vi "Point in Polygon_Classify Quadrant.vi"(6 "tolerance":dbl=1e-09, 8 "Polygon Y":dbl[](array[numeric]), 9 "Polygon X":dbl[](array[numeric]), 10 "y":dbl, 11 "x":dbl) -> (0 "vertex?":bool, 1 "Edge Angle":dbl[](array[numeric]), 2 "Edge Direct":dbl[](array[numeric]), 3 "Edge Quad":i16[](array[numeric]))   [LabVIEW 2020, in "NI_AAL_Geometry.lvlib"]
uses:
  <vilib>/Analysis/NI_AAL_Geometry.lvlib
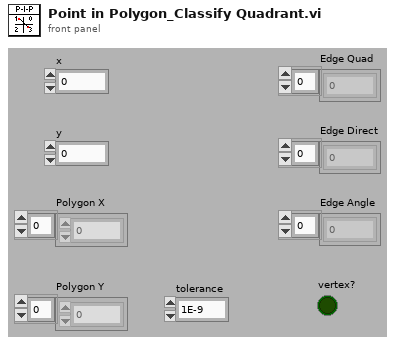
[diagram p1: front panel]
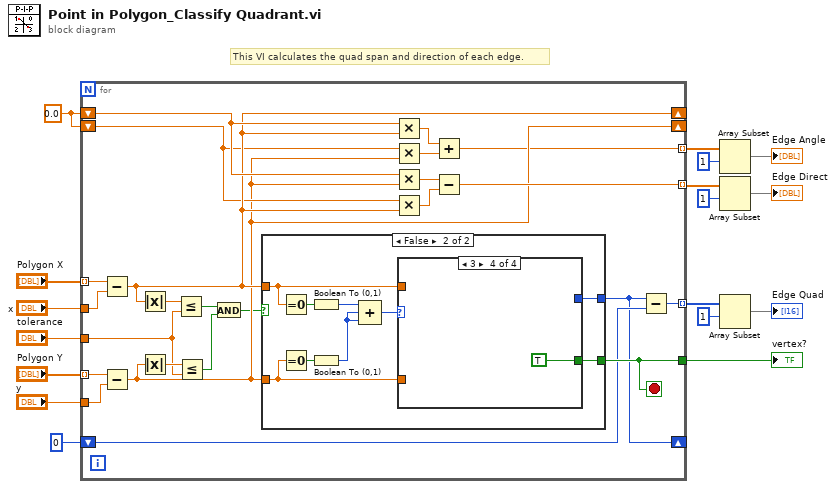
[diagram p0: block diagram]
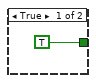
[diagram p2: hidden frame]
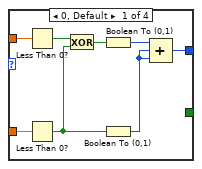
[diagram p3: hidden frame]
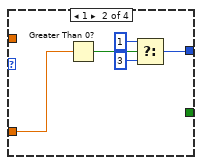
[diagram p4: hidden frame]
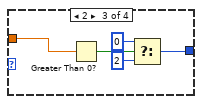
[diagram p5: hidden frame]
diagram:
  w5 = 0.0
  # "This VI calculates the quad span and direction of each edge."
  n1 = for {
    tunnel: "Polygon X" -> [w35] mode=indexing
    tunnel: "Polygon Y" -> [w40] mode=indexing
    tunnel: "x" -> [w41]
    tunnel: "y" -> [w39]
    tunnel: [w38] -> w13
    shift-right: [w18] -> _
    shift-left: i16 0 ("x") -> [w37]
    tunnel: [w36] -> w11 mode=indexing
    shift-right: [w27] -> _
    shift-left: w5 -> [w28]
    shift-right: [w25] -> _
    shift-left: w5 -> [w26]
    tunnel: [w33] -> w8 mode=indexing
    tunnel: "tolerance" -> [w30]
    tunnel: [w22] -> w2 mode=indexing
    stop <- w38 stop-if-true
    n2 = Subtract(x=w35, y=w41) -> (x-y=w27:dbl)
    n3 = Subtract(x=w40, y=w39) -> (x-y=w25:dbl)
    n4 = Absolute Value(x=w27) -> (abs(x)=w32:dbl)
    n5 = Absolute Value(x=w25) -> (abs(x)=w31:dbl)
    n6 = Less Or Equal?(x=w32, y=w30) -> (x <= y?=w21:bool)
    n7 = Less Or Equal?(x=w31, y=w30) -> (x <= y?=w20:bool)
    n8 = And(x=w21, y=w20) -> (x .and. y?=w19:bool)
    n9 = case shown="False" w19 {
      tunnel: [TRUE w51] -> w38
      tunnel: [_ w50] -> w18
      tunnel: w27 -> [_ w49]
      tunnel: w25 -> [_ w48]
      frame True {
      }
      frame False {
        n10 = Equal To 0?(x=w49) -> (x = 0?=w47:bool)
        n11 = Equal To 0?(x=w48) -> (x = 0?=w46:bool)
        n12 = Boolean To (0,1)(Boolean=w47) -> (0, 1=w45:i16)
        n13 = Boolean To (0,1)(Boolean=w46) -> (0, 1=w44:i16)
        n14 = Compound Arithmetic op=ADD(w45, w44, w44) -> (w43:i16)
        n15 = case shown="3" w43 {
          tunnel: w49 -> [w52 _ w68 _]
          tunnel: w48 -> [w59 w64 _ _]
          tunnel: [w58 w63 w69 _] -> w50
          tunnel: [_ _ _ TRUE] -> w51
          frame 0, Default {
            n16 = Less Than 0?(x=w52) -> (x < 0?=w57:bool)
            n17 = Less Than 0?(x=w59) -> (x < 0?=w54:bool)
            n18 = Exclusive Or(1:w54, 2:w57) -> (0:w55:bool)
            n19 = Boolean To (0,1)(Boolean=w55) -> (0, 1=w56:i16)
            n20 = Boolean To (0,1)(Boolean=w54) -> (0, 1=w53:i16)
            n21 = Compound Arithmetic op=ADD(w56, w53, w53) -> (w58:i16)
          }
          frame 1 {
            n22 = Greater Than 0?(x=w64) -> (x > 0?=w62:bool)
            n23 = Select(t=i16 1, s=w62, f=i16 3) -> (s? t:f=w63:i16)
          }
          frame 2 {
            n24 = Greater Than 0?(x=w68) -> (x > 0?=w67:bool)
            n25 = Select(t=i16 0, s=w67, f=i16 2) -> (s? t:f=w69:i16)
          }
          frame 3 {
          }
        }
      }
    }
    n26 = Multiply(x=w28, y=w27) -> (x*y=w24:dbl)
    n27 = Multiply(x=w26, y=w25) -> (x*y=w23:dbl)
    n28 = Multiply(x=w28, y=w25) -> (x*y=w29:dbl)
    n29 = Multiply(x=w26, y=w27) -> (x*y=w34:dbl)
    n30 = Add(x=w24, y=w23) -> (x+y=w22:dbl)
    n31 = Subtract(x=w29, y=w34) -> (x-y=w33:dbl)
    n32 = Subtract(x=w18, y=w37) -> (x-y=w36:i16)
  }
  "vertex?" <- w13
  n33 = Array Subset(array=w2, index=1) -> (→"Edge Angle":dbl[])  [unwired: 1 in]
  n34 = Array Subset(array=w8, index=1) -> (→"Edge Direct":dbl[])  [unwired: 1 in]
  n35 = Array Subset(array=w11, index=1) -> (→"Edge Quad":i16[])  [unwired: 1 in]
